vi "Acquire Digital.vi"(8 "error in (no error)":errorcluster, 11 "Digital Input in":refnum<class "Digital Input.lvclass">) -> (0 "error out":errorcluster, 3 "Digital Input out":refnum<class "Digital Input.lvclass">)   [LabVIEW 2021, in "Digital Input.lvlib" / "Digital Input.lvclass"]
uses:
  Digital Input.lvclass
  C:/Program Files/National Instruments/LabVIEW 2021/vi.lib/ActorFramework/Actor/Actor.lvclass
  <vilib>/ActorFramework/Actor/Actor.lvclass/Actor.ctl
  <vilib>/ActorFramework/Message Enqueuer/Message Enqueuer.lvclass/Message Enqueuer.ctl
  Digital Input.lvclass/Digital Input.ctl
  <vilib>/DAQmx/read.llb/DAQmx Read (Digital 1D Wfm NChan NSamp).vi
  <vilib>/ActorFramework/Message Enqueuer/Init from Existing Queue.vi
  <vilib>/ActorFramework/Message Enqueuer/Enqueue.vi
  Digital Input Messages/Acquire Digital Msg/Acquire Digital Msg.lvclass
  C:/Program Files/National Instruments/LabVIEW 2021/vi.lib/ActorFramework/Message/Message.lvclass
  <vilib>/ActorFramework/Message Priority Queue/Priority Enqueue.vi
  <vilib>/DAQmx/miscellaneous.llb/DAQmx Fill In Error Info.vi
  <vilib>/ActorFramework/Message Enqueuer/Message Enqueuer.lvclass
  <vilib>/ActorFramework/Actor/Actor.lvclass
  C:/git/Digital-Tasks/Digital Input/Digital Input/Digital Input/Digital Input.lvclass
  Digital Input Interface Messages/Digital Input Interface Messages Messages/Digital Input Signals Msg/Digital Input Signals Msg.lvclass
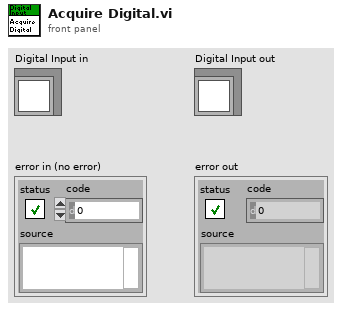
[diagram p1: front panel]
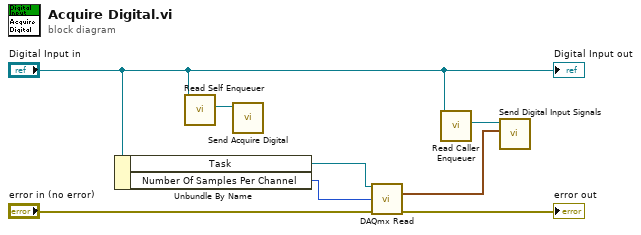
[diagram p0: block diagram]
diagram:
  n1 = Unbundle By Name("Digital Input in") -> ("Task"=w6:refnum<k21>, "Number Of Samples Per Channel"=w5:i32)
  n2 = call <vilib>:"Read Self Enqueuer.vi"("Actor"="Digital Input in") -> ("Self Enqueuer"=w3:refnum<class "Message Enqueuer.lvclass">)  [unwired: 10 in]
  n3 = call "Send Acquire Digital.vi"("Message Enqueuer"=w3) -> ()  [unwired: 9 in, 2 out]
  n4 = call-poly <vilib>:"DAQmx Read.vi"("task/channels in"=w6, "number of samples per channel"=w5, "error in"="error in (no error)") -> ("data"=w1:digitalwaveform[], "error out"=→"error out":errorcluster)  [unwired: 10 in, 1 out]
  n5 = call <vilib>:"Read Caller Enqueuer.vi"("Actor"="Digital Input in") -> ("Caller Enqueuer"=w2:refnum<class "Message Enqueuer.lvclass">)  [unwired: 10 in]
  n6 = call "Send Digital Input Signals.vi"("Digital Input Signals"=w1, "Message Enqueuer"=w2) -> ()  [unwired: 8 in, 2 out]
  "Digital Input out" <- "Digital Input in"
